vi "p02operaciones.vi"() -> ()   [LabVIEW 2013]
panel:
  in  "Vertical Pointer Slide":dbl(slide) scale=0.0..10.0
  out "Waveform Graph":dbl[][](graph)
  out "2D Picture 2":picture
  out "2D Picture":picture
  in  "path to BMP file":path
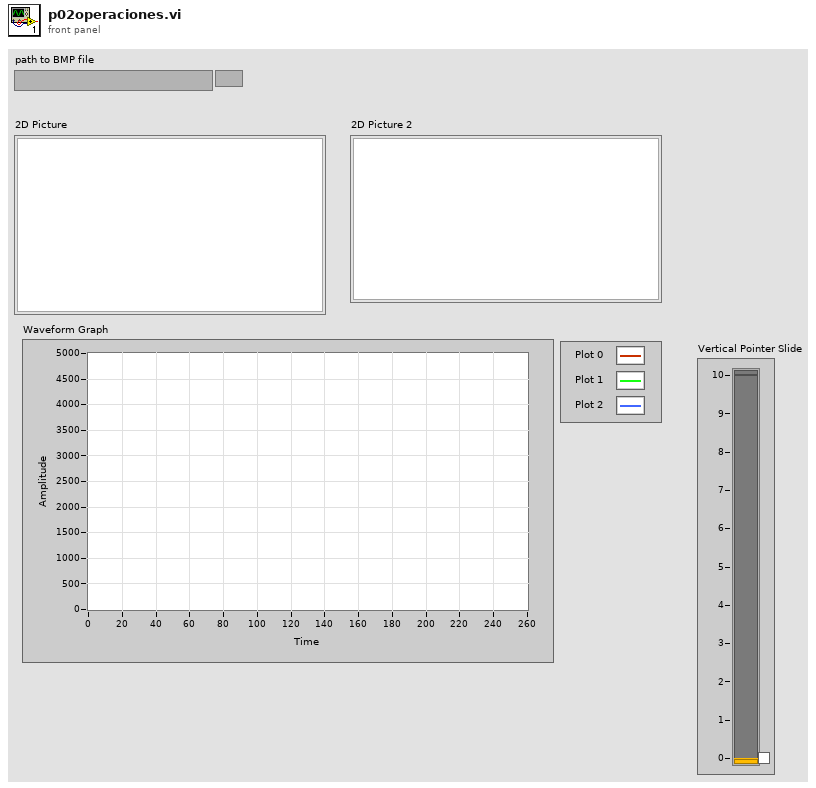
[diagram p1: front panel]
types:
  T1 = typedef "imagedata.ctl" = cluster{"image type":i32, "image depth":i32, "image":u8[], "mask":u8[], "colors":u32[], "Rectangle":cluster{"left":i16, "top":i16, "right":i16, "bottom":i16}}
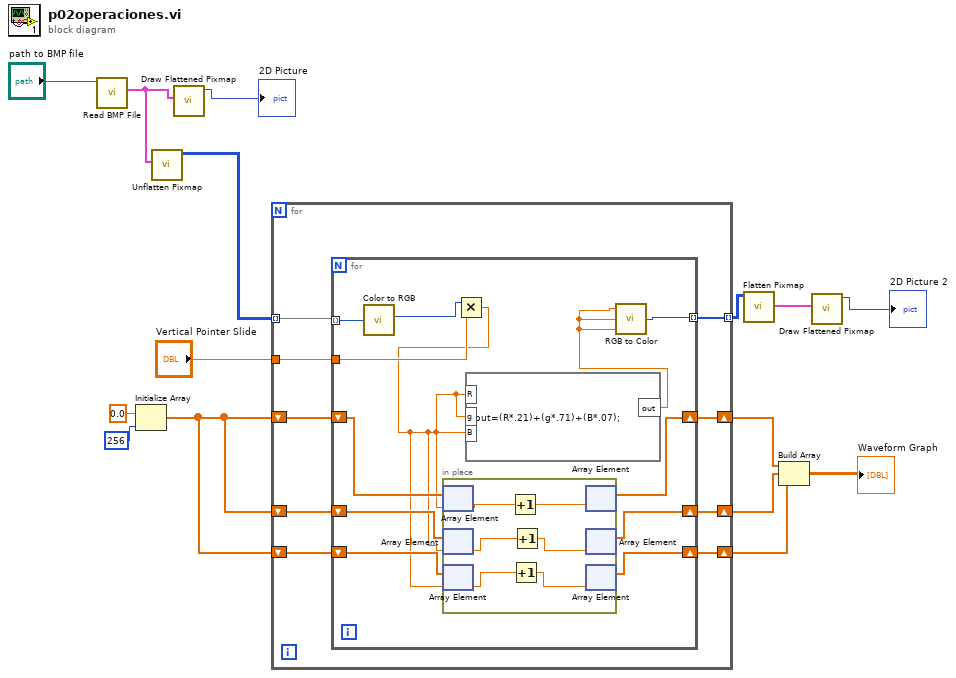
[diagram p0: block diagram]
diagram:
  n1 = call <vilib>:"Read BMP File.vi"("path to BMP file"="path to BMP file") -> ("image data"=w13:T1)  [unwired: 8 in, 2 out]
  n2 = Initialize Array(0.0 ("element"), 256 ("dimension size")) -> (w6:dbl[])
  n3 = call <vilib>:"Unflatten Pixmap.vi"("image data"=w13) -> ("24-bit pixmap"=w12:u32[][])  [unwired: 4 in, 6 out]
  n4 = call <vilib>:"Draw Flattened Pixmap.vi"("image data"=w13) -> ("new picture"=→"2D Picture":picture)  [unwired: 8 in]
  n5 = for {
    tunnel: w12 -> [w24] mode=indexing
    tunnel: [w23] -> w11 mode=indexing
    shift-right: [w21] -> w5
    shift-left: w6 -> [w22]
    shift-right: [w18] -> w4
    shift-left: w6 -> [w20]
    shift-right: [w17] -> w3
    shift-left: w6 -> [w19]
    tunnel: "Vertical Pointer Slide" -> [w16]
    n6 = for {
      tunnel: w24 -> [w36] mode=indexing
      tunnel: [w35] -> w23 mode=indexing
      shift-right: [w32] -> w21
      shift-left: w22 -> [w33]
      shift-right: [w29] -> w18
      shift-left: w20 -> [w31]
      shift-right: [w28] -> w17
      shift-left: w19 -> [w30]
      tunnel: w16 -> [w26]
      n7 = call <vilib>:"Color to RGB.vi"("Color"=w36) -> ("R"=w27:u8)  [unwired: 3 out]
      n8 = Multiply(x=w27, y=w26) -> (x*y=w25:dbl)
      n9 = in-place {
        n10 = in-place-array #1(w33, w25) -> (w42:dbl)
        n11 = in-place-array #2(w31, w25) -> (w40:dbl)
        n12 = in-place-array #3(w30, w25) -> (w39:dbl)
        n13 = Increment(x=w42) -> (x+1=w41:dbl)
        n14 = Increment(x=w39) -> (x+1=w37:dbl)
        n15 = Increment(x=w40) -> (x+1=w38:dbl)
        n16 = in-place-array #1(w41) -> (w32:dbl[])  [unwired: 1 out]
        n17 = in-place-array #2(w38) -> (w29:dbl[])  [unwired: 1 out]
        n18 = in-place-array #3(w37) -> (w28:dbl[])  [unwired: 1 out]
      }
      n19 = formula code="out=(R*.21)+(g*.71)+(B*.07);"("R"=w25, "B"=w25, "g"=w25) -> ("out"=w34:dbl)
      n20 = call <vilib>:"RGB to Color.vi"("B"=w34, "G"=w34, "R"=w34) -> ("Color"=w35:u32)
    }
  }
  n21 = call <vilib>:"Flatten Pixmap.vi"("24-bit pixmap"=w11) -> ("image data"=w10:T1)  [unwired: 10 in]
  n22 = Build Array(w5, w4, w3) -> (→"Waveform Graph":dbl[][])
  n23 = call <vilib>:"Draw Flattened Pixmap.vi"("image data"=w10) -> ("new picture"=→"2D Picture 2":picture)  [unwired: 8 in]
